vi "ViewRunInfo.vi"(11 "Run Info In":T1={"Active Run?"=FALSE, "Run Notes"="Enter in notes explaining the purpose of the run and any unusual steps taken in the process. This note should make it clear *why* you are taking data. More specifically, you should record information about any changes to the system that were made OUTSIDE of LabView.  There is no way to automatically record such changes, so it is up to you to describe it here (or else the data will be useless!) .\n\nAfter such changes is also precisely when you should start a new run. For example, if you changed to using the solicited trigger, if you changed the amount of LXe in the cell, etc. There are no other reasons to start a new run. Do not start a new run just because you changed a setting inside LabView. Doing so will over-fragment data and cause clutter, making it more difficult to actually do physics with it later.\n\nThank You\n- Reed Cohen", "User Name"="", "Campaign ID#"="", "Run Name"="", "Start Time"=timestamp(0 s since 1904-01-01), "End Time"=timestamp(0 s since 1904-01-01)}) -> ()   [LabVIEW 2012]
uses:
  TypeDefs/DataTypes/RunInfo.ctl
panel:
  in  "OK Button":bool
  out "Campaign ID#":string
  out "Run Name":string
  out "User Name":string
  out "Run Notes":string="Enter in notes explaining the purpose of the run and any unusual steps taken in the process. This note should make it clear *why* you are taking data. More specifically, you should record information about any changes to the system that were made OUTSIDE of LabView.  There is no way to automatically record such changes, so it is up to you to describe it here (or else the data will be useless!) .\n\nAfter such changes is also precisely when you should start a new run. For example, if you changed to using the solicited trigger, if you changed the amount of LXe in the cell, etc. There are no other reasons to start a new run. Do not start a new run just because you changed a setting inside LabView. Doing so will over-fragment data and cause clutter, making it more difficult to actually do physics with it later.\n\nThank You\n- Reed Cohen"
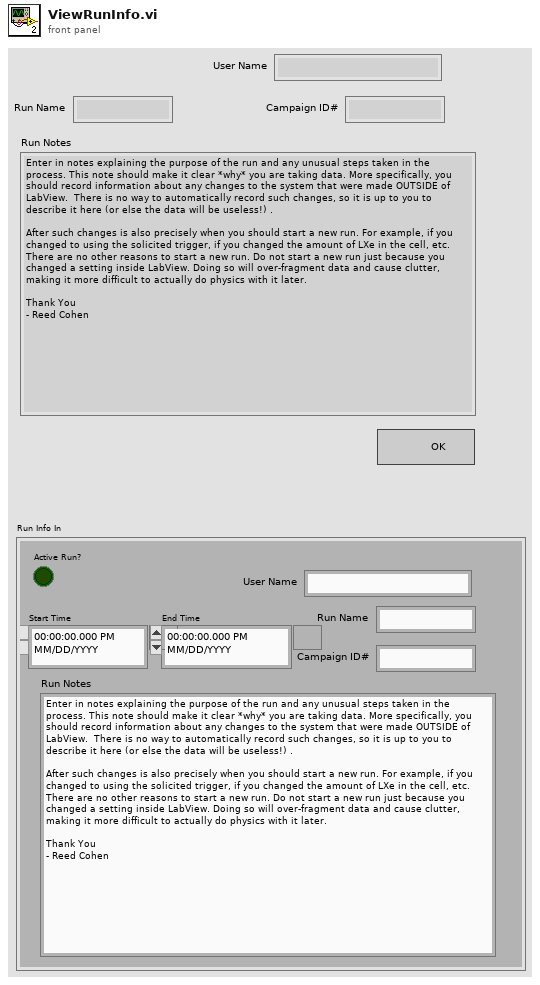
[diagram p1: front panel]
types:
  T1 = typedef "RunInfo.ctl" = cluster{"Active Run?":bool, "Run Notes":string, "User Name":string, "Campaign ID#":string, "Run Name":string, "Start Time":timestamp, "End Time":timestamp}
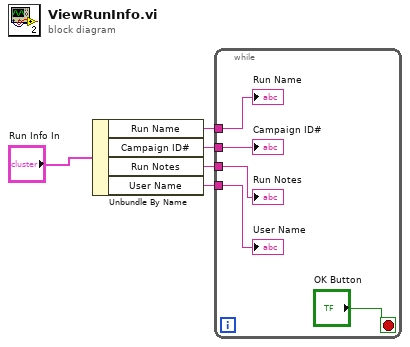
[diagram p0: block diagram]
diagram:
  n1 = Unbundle By Name("Run Info In") -> ("Run Name"=w1:string, "Campaign ID#"=w2:string, "Run Notes"=w3:string, "User Name"=w4:string)
  n2 = while {
    tunnel: w4 -> [w9]
    tunnel: w3 -> [w8]
    tunnel: w2 -> [w7]
    tunnel: w1 -> [w6]
    stop <- "OK Button" stop-if-true
    "Run Notes" <- w8
    "User Name" <- w9
    "Run Name" <- w6
    "Campaign ID#" <- w7
  }
